vi "QDInstrument_Example_Simple.vi"() -> ()   [LabVIEW 2019]
panel:
  out "ISO8601 UTC DateTime":string
  out "Temperature":dbl
  in  "stop":bool
  in  "IP Address":string="localhost"
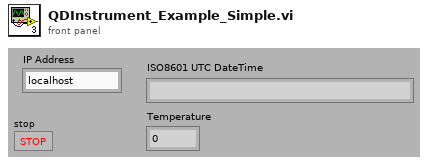
[diagram p1: front panel]
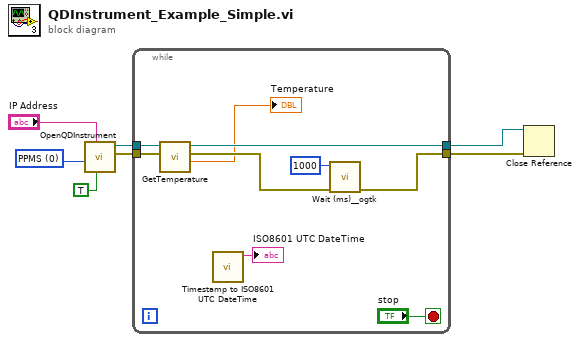
[diagram p0: block diagram]
diagram:
  w6 = 0 items=["PPMS", "VersaLab", "DynaCool", "SVSM"] ("Instrument\nType")
  n1 = call "OpenQDInstrument.vi"("Remote"=TRUE, "IP Address"="IP Address", "Instrument Type"=w6) -> ("error out"=w3:errorcluster, "Instrument Ref"=w4:refnum<k24>)  [unwired: 5 in]
  n2 = while {
    tunnel: w4 -> [w16]
    tunnel: w3 -> [w15]
    tunnel: [w14] -> w2
    tunnel: [w12] -> w1
    stop <- "stop" stop-if-true
    n3 = call "GetTemperature.vi"("error in (no error)"=w15, "Instrument Ref In"=w16) -> ("Temperature"=→"Temperature":dbl, "error out"=w13:errorcluster, "Instrument Ref Out"=w14:refnum<k24>)  [unwired: 3 in, 2 out]
    n4 = call <vilib>:"Timestamp to ISO8601 UTC DateTime.vi"() -> ("ISO8601 UTC DateTime"=→"ISO8601 UTC DateTime":string)  [unwired: 11 in]
    n5 = call <userlib>:"Wait (ms)__ogtk.vi"("error in (no error)"=w13, "milliseconds to wait"=u32 1000) -> ("error out"=w12:errorcluster)  [unwired: 8 in, 1 out]
  }
  n6 = Close Reference(reference=w2, error in (no error)=w1) -> ()  [unwired: 1 out]
